vi "Ring selection test.vi"(8 "error in (no error)":errorcluster, 11 "RSA in":refnum<class "RSA.lvclass">) -> (0 "error out":errorcluster, 3 "RSA out":refnum<class "RSA.lvclass">)   [LabVIEW 2012, in "RSA.lvclass"]
uses:
  RSA.lvclass
  <vilib>/Analysis/NI_AALBase.lvlib
panel:
  out "Histogram Graph":T1(graph)
  in  "Numeric":i32
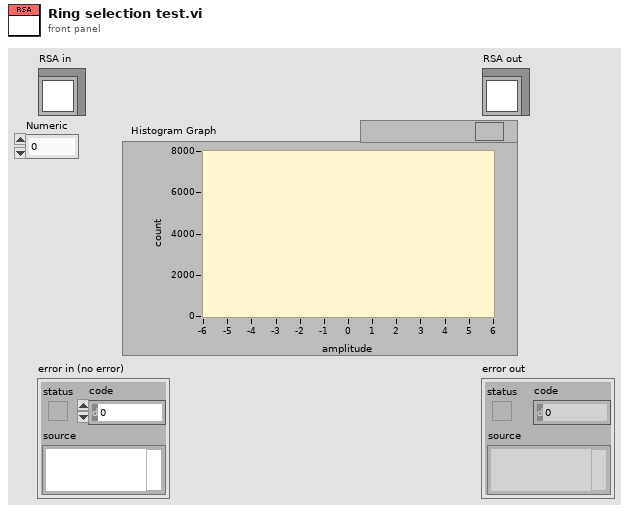
[diagram p1: front panel]
types:
  T1 = cluster{"X Values":dbl[], "Histogram: h(x)":i32[]}
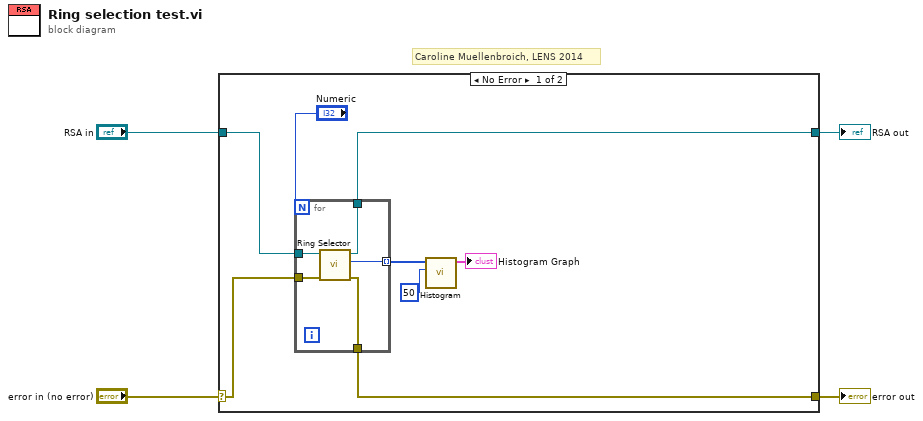
[diagram p0: block diagram]
diagram:
  # "Caroline Muellenbroich, LENS 2014"
  n1 = case shown="No Error" "error in (no error)" {
    selector: "error in (no error)" -> [w10 w18]
    tunnel: [w9 w18] -> w1
    tunnel: [w11 w19] -> w2
    tunnel: "RSA in" -> [w12 w19]
    frame No Error {
      n2 = for {
        N: "Numeric" -> [_]
        tunnel: w12 -> [w17]
        tunnel: [w16] -> w11
        tunnel: w10 -> [w15]
        tunnel: [w14] -> w9
        tunnel: [w13] -> w7 mode=indexing
        n3 = call-dynamic "Ring Selector.vi"("error in (no error)"=w15, "RSA in"=w17) -> ("error out"=w14:errorcluster, "Ringnumber"=w13:i32, "RSA out"=w16:refnum<class "RSA.lvclass">)  [unwired: 7 in]
      }
      n4 = call <vilib>:"Histogram.vi"("intervals"=50, "X"=w7) -> ("Histogram Graph"=→"Histogram Graph":T1)  [unwired: 6 in, 3 out]
    }
    frame Error {
    }
  }
  "error out" <- w1
  "RSA out" <- w2
